vi "SnoUpdateAutoCommandFileNames.vi"(1 "error in (no error)":errorcluster) -> (0 "error out":errorcluster, 2 "filenames":string[](array[string]))   [LabVIEW 2014]
uses:
  <vilib>/Rock Robotics/Network Tables/SD Write String.vi
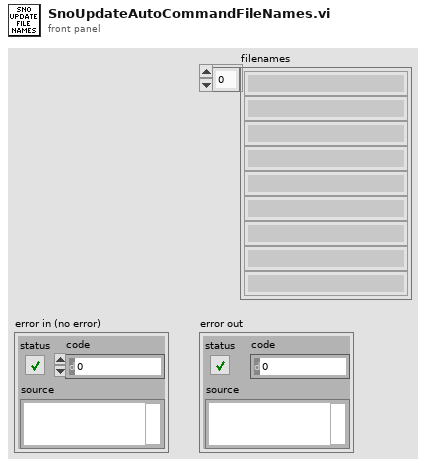
[diagram p1: front panel]
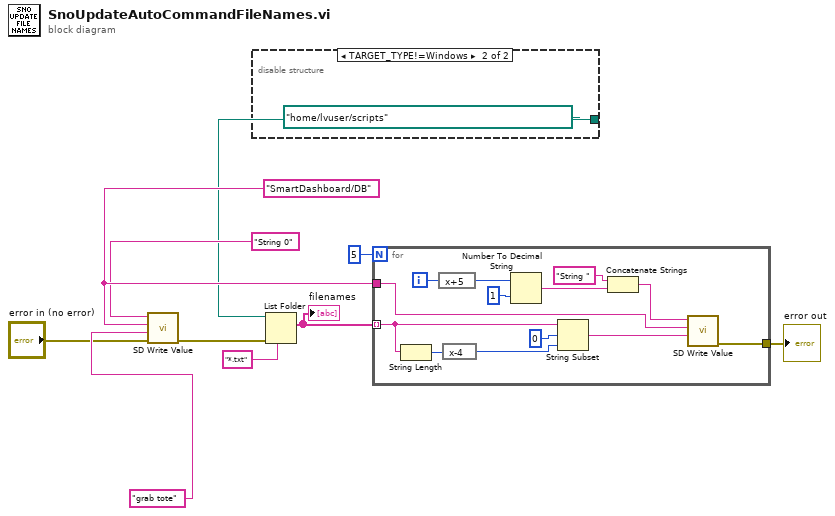
[diagram p0: block diagram]
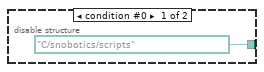
[diagram p2: hidden frame]
diagram:
  w7 = "SmartDashboard/DB" ("Table Prefix")
  n1 = call-poly <vilib>:"SD Write Value.vi"("error in"="error in (no error)", "String"="grab tote" ("Name"), "Table Prefix"=w7, "Name"="String 0") -> ("error out"=w9:errorcluster)  [unwired: 6 in, 1 out]
  n2 = disable-structure shown="TARGET_TYPE!=Windows" {
    disable-tunnel: [path "C:/snobotics/scripts" ("path") path "/home/lvuser/scripts" ("Simulator Script Name")] -> w3
    frame condition #0 {
    }
    frame condition #1 (active) {
    }
  }
  n3 = List Folder(path=w3, pattern="*.txt", error in=w9) -> (filenames=w4:string[])  [unwired: 1 in, 3 out]
  "filenames" <- w4
  n4 = for {
    N: 5 -> [_]
    tunnel: w4 -> [w16] mode=indexing
    tunnel: w7 -> [w25]
    tunnel: [w20] -> w5
    i -> [w23]
    n5 = String Length(string=w16) -> (length=w15:i32)
    n6 = expression code="x+5"(w23) -> (w21:i32)
    n7 = expression code="x-4"(w15) -> (w14:i32)
    n8 = Number To Decimal String(number=w21, width (-)=i16 1) -> (decimal integer string=w24:string)
    n9 = String Subset(string=w16, offset (0)=0, length (rest)=w14) -> (substring=w13:string)
    n10 = Concatenate Strings("String ", w24) -> (w19:string)
    n11 = call-poly <vilib>:"SD Write Value.vi"("String"=w13, "Table Prefix"=w25, "Name"=w19) -> ("error out"=w20:errorcluster)  [unwired: 7 in, 1 out]
  }
  "error out" <- w5
